vi "Load Type Images.vi"(11 "data type":string) -> (0 "bottom":T1, 1 "value":T1, 2 "header":T1, 3 "single":T1)   [LabVIEW 2015, in "Build JSON Array.xnode"]
uses:
  Build JSON Array.xnode
  <vilib>/picture/picture.llb/imagedata.ctl
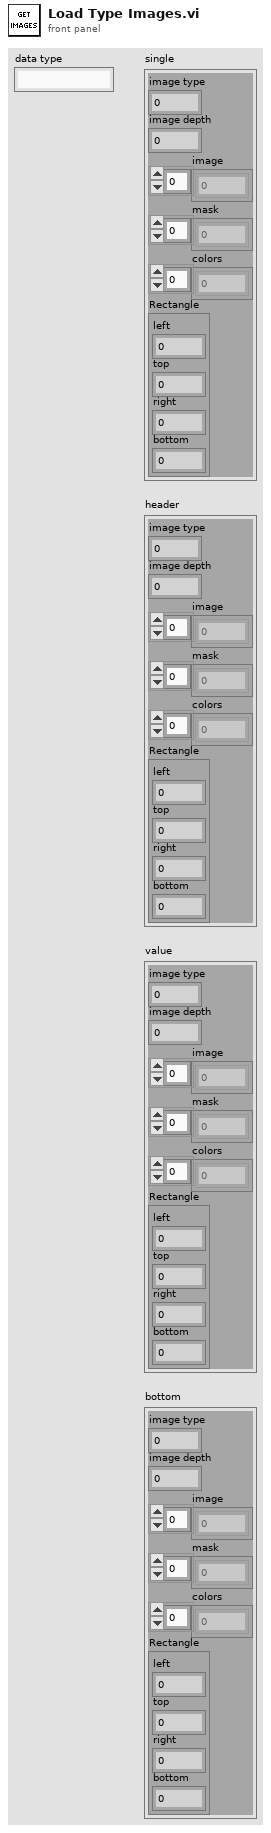
[diagram p1: front panel]
types:
  T1 = typedef "imagedata.ctl" = cluster{"image type":i32, "image depth":i32, "image":u8[], "mask":u8[], "colors":u32[], "Rectangle":cluster{"left":i16, "top":i16, "right":i16, "bottom":i16}}
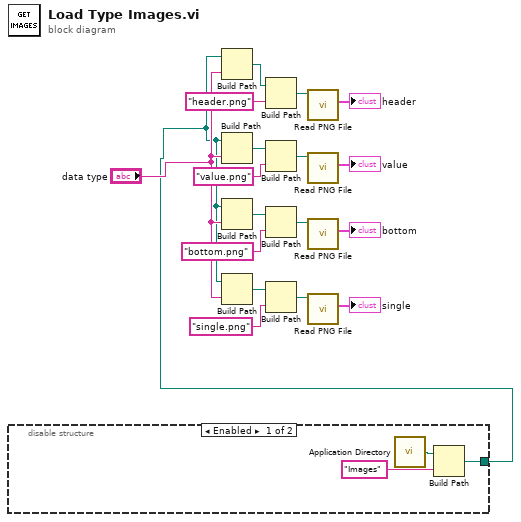
[diagram p0: block diagram]
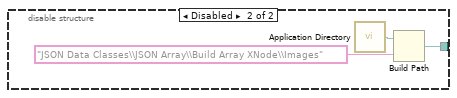
[diagram p2: hidden frame]
diagram:
  n1 = disable-structure shown="Enabled" {
    disable-tunnel: [w20 w23] -> w1
    frame Enabled {
      n2 = call <vilib>:"Application Directory.vi"() -> ("Application Directory"=w19:path)
      n3 = Build Path(base path=w19, name or relative path="Images") -> (appended path=w20:path)
    }
    frame Disabled {
      n4 = call <vilib>:"Application Directory.vi"() -> ("Application Directory"=w22:path)
      n5 = Build Path(base path=w22, name or relative path="JSON Data Classes\\JSON Array\\Build Array XNode\\Images") -> (appended path=w23:path)
    }
  }
  n6 = Build Path(base path=w1, name or relative path="data type") -> (appended path=w3:path)
  n7 = Build Path(base path=w1, name or relative path="data type") -> (appended path=w4:path)
  n8 = Build Path(base path=w1, name or relative path="data type") -> (appended path=w5:path)
  n9 = Build Path(base path=w1, name or relative path="data type") -> (appended path=w2:path)
  n10 = Build Path(base path=w3, name or relative path="header.png") -> (appended path=w12:path)
  n11 = Build Path(base path=w4, name or relative path="value.png") -> (appended path=w13:path)
  n12 = Build Path(base path=w5, name or relative path="bottom.png") -> (appended path=w14:path)
  n13 = Build Path(base path=w2, name or relative path="single.png") -> (appended path=w11:path)
  n14 = call <vilib>:"Read PNG File.vi"("path to PNG file"=w12) -> ("image data"=→"header":T1)  [unwired: 8 in, 2 out]
  n15 = call <vilib>:"Read PNG File.vi"("path to PNG file"=w13) -> ("image data"=→"value":T1)  [unwired: 8 in, 2 out]
  n16 = call <vilib>:"Read PNG File.vi"("path to PNG file"=w14) -> ("image data"=→"bottom":T1)  [unwired: 8 in, 2 out]
  n17 = call <vilib>:"Read PNG File.vi"("path to PNG file"=w11) -> ("image data"=→"single":T1)  [unwired: 8 in, 2 out]
